vi "pco.camera_Live_Example_IMAQ.vi"() -> ()   [LabVIEW 2020]
doc: "A short program to demonstrate the fundamentals of control and image acquision with the pco.camera series. The program records a sequence of images, with \"live\" updating, until the \"StopRecording\" button is pressed. Use ctrl-H for more help on the individual controls and indicators.\n\nCopyright 2004, 2010 The Cooke Corporation."
uses:
  <userlib>/PCO LabVIEW 5.0.0/pco.camera/Camera.lvclass
  <userlib>/PCO LabVIEW 5.0.0/pco.sdk/TimingControl/TimingControl.lvlib
panel:
  in  "Trigger":bool
  in  "data_format":T1(ring)=enum."Mono16"
  out "Image":T2(plugin-control)
  out "rawImage":u16[][](array[numeric])
  in  "Image Index":u32 max=9
  out "Recorded Images":u32
  in  "TriggerMode":T3(ring)
  in  "Quit":bool
  out "Error":errorcluster {"code" format="%x"}
  in  "Stop Record":bool
  out "Recording On":bool
  in  "roiY1":u64=2 min=1 max=2160 step=1
  in  "roiX1":u64=2 min=1 max=2560 step=1
  in  "roiY0":u64=1 min=1 max=2159 step=1
  in  "roiX0":u64=1 min=1 max=2559 step=1
  out "Image Height":u64
  out "Image Width":u64
  in  "dwImgCount":u32=10 caption="Required Number of Images" max=2397
  in  "Exposure Time [s]":dbl=0.010000000000000002 min=0.0005 max=2.0 step=0.001
  # "This example demonstrates the image acquisition with one camera in ring buffer mode together with a live display of the latest images during record. After record is stopped, the images can be addressed by index.\nNote that this example will not be fail save, i.e. doesnt react on errors, just handles them forward to the end\n\nUsage:\nSelect your required image count, data format and the camera setup before you start the program.\nOnce started, the camera class will be initialized and images will be recorded and displayed automatically\nYou can stop the images by pressing stop record.\nAfter stopped, the image at the selected index will be read out\nTo finish the program click on quit application, this will force an exit of the camera class\nYou can change your required ROI after and also during the record."
  # "pco.labview"
  # "Camera Setup"
  # "Recording Control"
  # "Parameters for image readout"
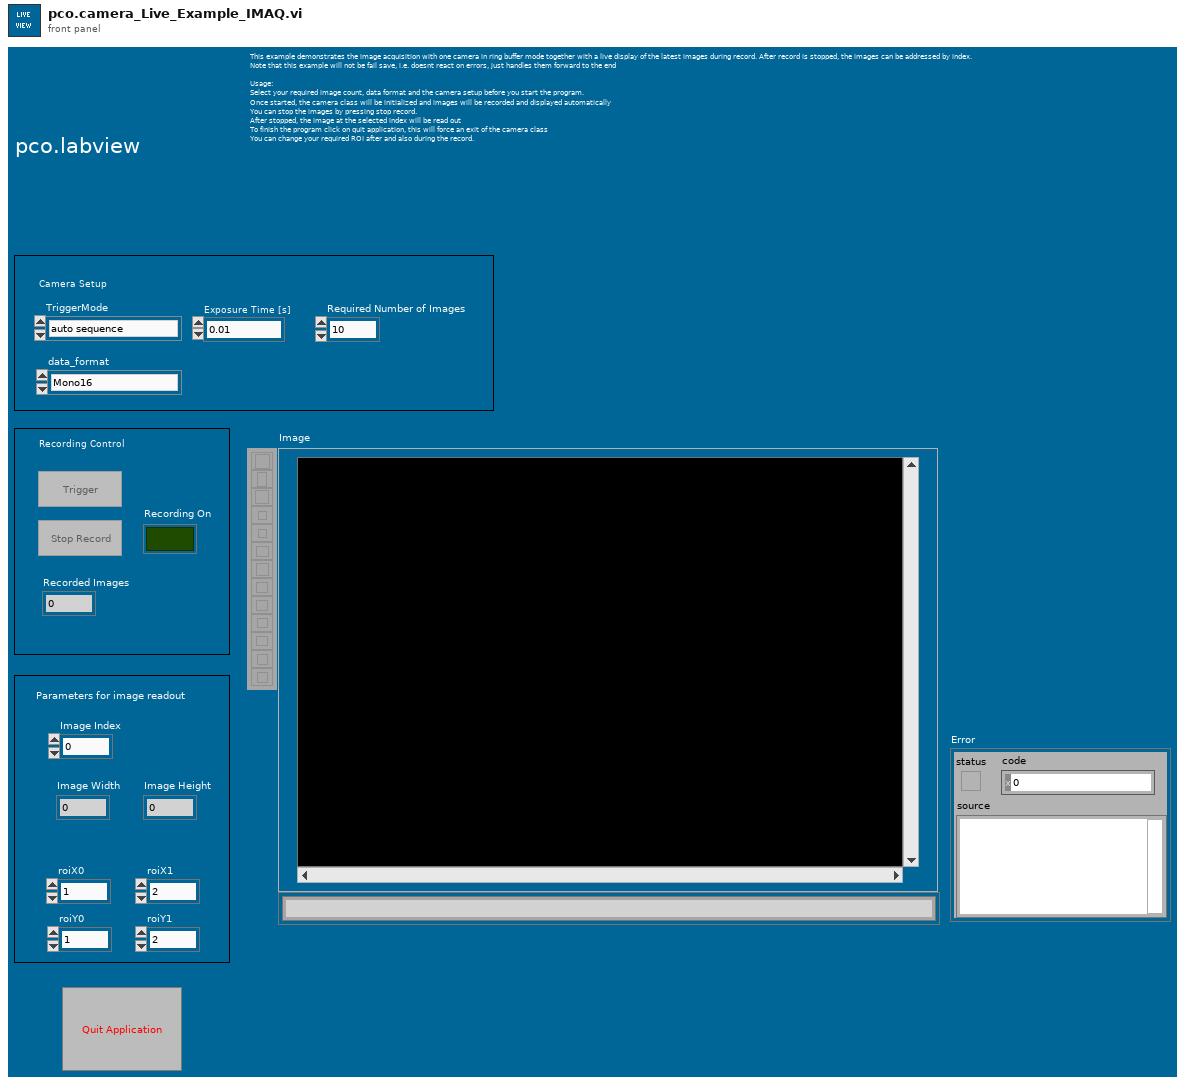
[diagram p1: front panel]
types:
  T1 = enum16{"Undefined", "Mono8", "Mono16", "BGRA8", "RGBA8", "BGRA16", "RGBA16", "CompressedMono8"}
  T2 = typedef "IMAQ Image.ctl" = refnum<image>
  T3 = enum16{"auto sequence", "software trigger", "external exposure start", "external exposure control"}
  T4 = enum16{"sequence", "sequence non blocking", "ring buffer", "fifo", "sequence_dpcore", "sequence_non_blocking_dpcore", "ring_buffer_dpcore", "fifo_dpcore", "tif", "multitif", "pcoraw", "b16", "dicom", "multidicom"}
  T5 = enum8{"Enabled", "Disabled", "Disabled and Grayed Out"}
  T6 = cluster{"serial":u32, "type":u16, "sub_type":u16, "interface_type":u16, "min_exposure_time_s":dbl, "max_exposure_time_s":dbl, "min_exposure_step_s":dbl, "min_delay_time_s":dbl, "max_delay_time_s":dbl, "min_delay_step_s":dbl, "min_width":u64, "min_height":u64, "max_width":u64, "max_height":u64, "roi_step_horz":u64, "roi_step_vert":u64, "roi_symmetric_horz":bool, "roi_symmetric_vert":bool, "has_timestamp_mode":bool, "has_timestamp_mode_ascii_only":bool, "pixelrate_vec":u32[], "has_acquire_mode":bool, "has_ext_acquire_mode":bool, "has_metadata_mode":bool, "has_ram":bool, "binning_horz_vec":u16[], "binning_vert_vec":u16[]}
  T7 = typedef "Image Type" = u32
  T8 = typedef "Camera.lvclass/binning.ctl" = cluster{"vert":u16, "horz":u16}
  T9 = cluster{"exposure_time_s":dbl, "delay_time_s":dbl, "roi":cluster{"x0":u64, "y0":u64, "x1":u64, "y1":u64}, "timestamp_mode":u16, "pixelrate":u32, "trigger_mode":u16, "acquire_mode":u16, "metadata_mode":u16, "noisefilter_mode":u16, "binning":T8}
  T10 = typedef "Color (U64)" = cluster{"Plane 3 (Blue)":u16, "Plane 2 (Green)":u16, "Plane 1 (Red)":u16, "Plane 4 (alpha)":u16}
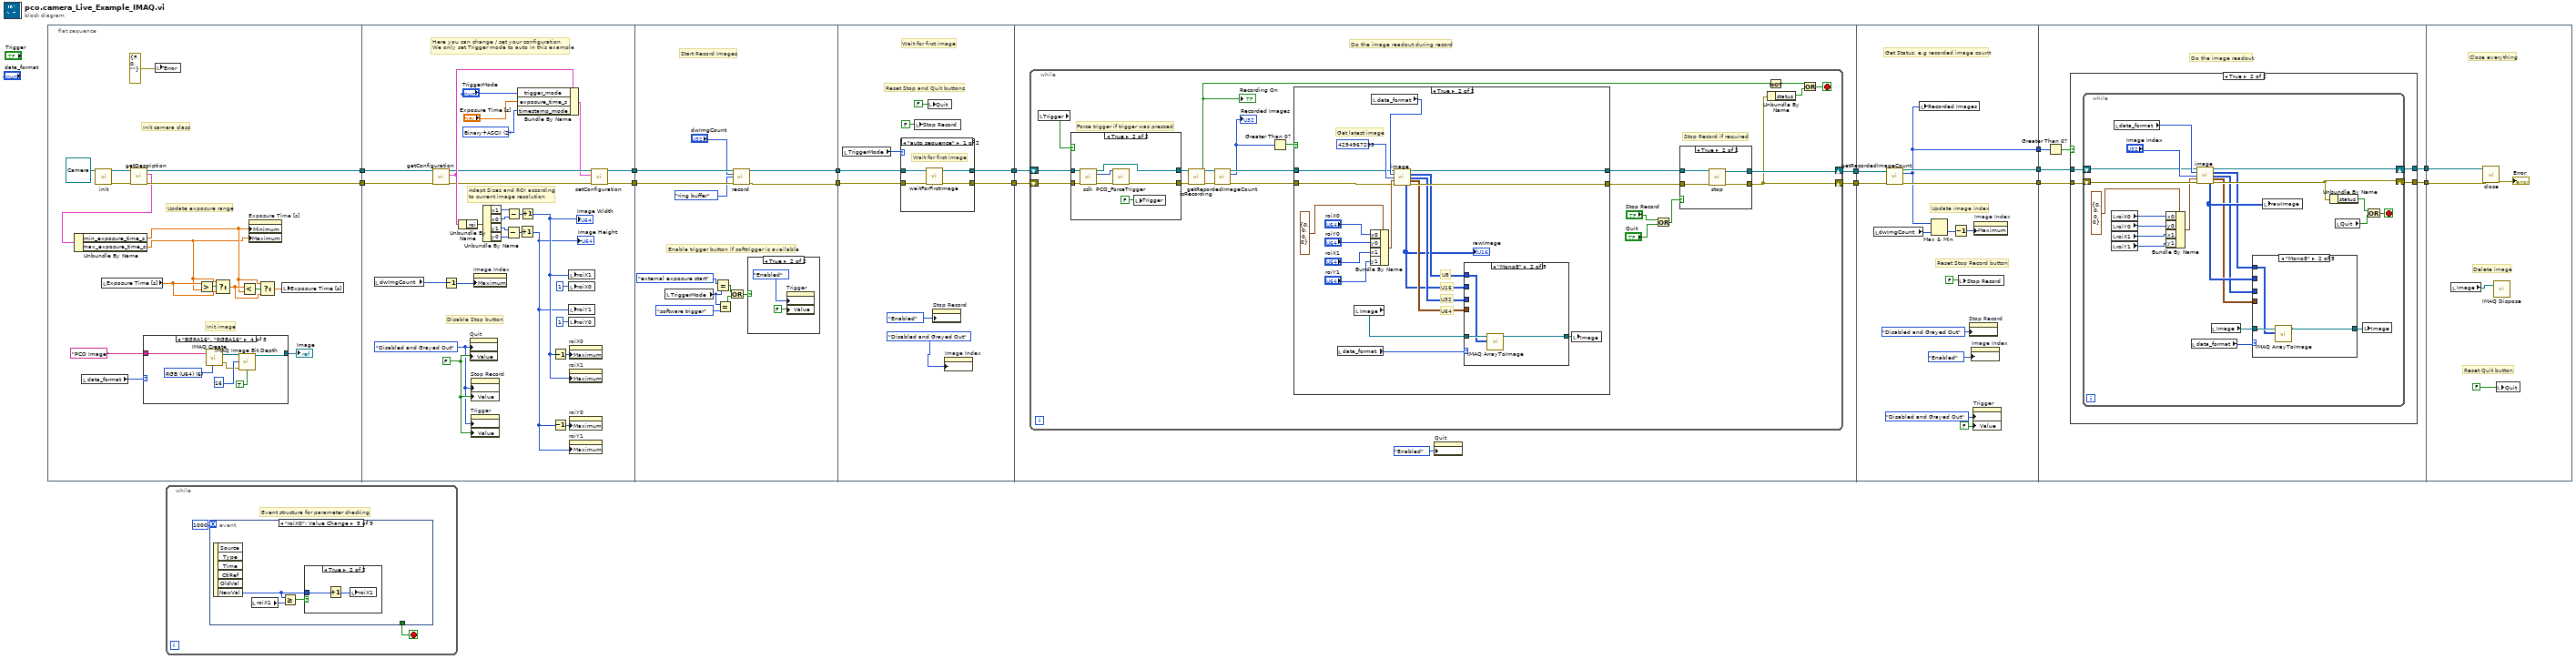
[diagram p0: block diagram]
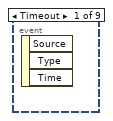
[diagram p2: hidden frame]
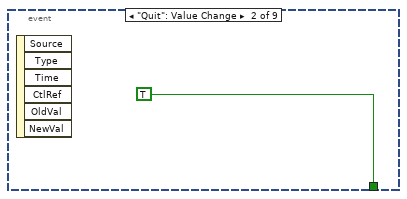
[diagram p3: hidden frame]
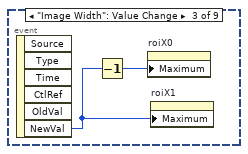
[diagram p4: hidden frame]
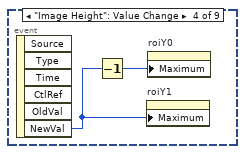
[diagram p5: hidden frame]
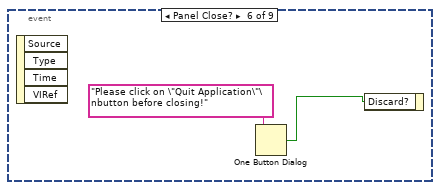
[diagram p7: hidden frame]
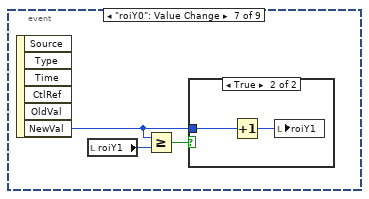
[diagram p8: hidden frame]
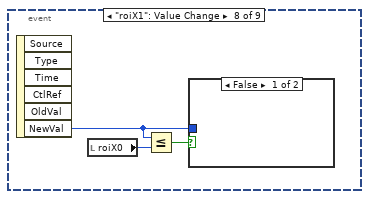
[diagram p10: hidden frame]
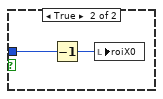
[diagram p11: hidden frame]
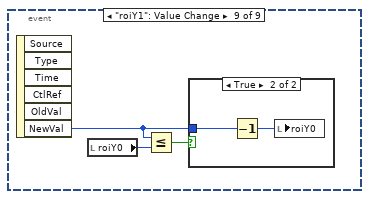
[diagram p12: hidden frame]
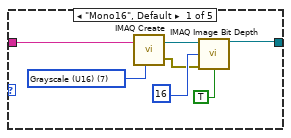
[diagram p14: hidden frame]
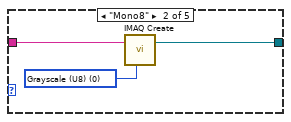
[diagram p15: hidden frame]
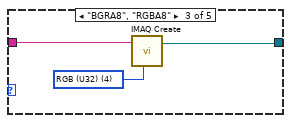
[diagram p16: hidden frame]
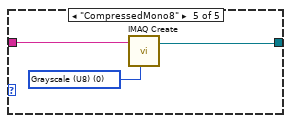
[diagram p17: hidden frame]
diagram:
  n1 = flat-sequence {
    tunnel: [w21] -> w7
    tunnel: [w20] -> w6
    tunnel: [w60] -> w15
    tunnel: [w64] -> w14
    tunnel: w7 -> [w59]
    tunnel: w6 -> [w58]
    tunnel: [w84] -> w9
    tunnel: [w85] -> w8
    tunnel: w14 -> [w95]
    tunnel: w15 -> [w94]
    tunnel: w9 -> [w102]
    tunnel: w8 -> [w103]
    tunnel: [w101] -> w13
    tunnel: [w99] -> w2
    tunnel: w13 -> [w117]
    tunnel: [w115] -> w12
    tunnel: [w114] -> w5
    tunnel: w2 -> [w113]
    tunnel: w12 -> [w200]
    tunnel: [w198] -> w11
    tunnel: w5 -> [w193]
    tunnel: [w192] -> w4
    tunnel: [w191] -> w1
    tunnel: w11 -> [w209]
    tunnel: [w208] -> w10
    tunnel: w4 -> [w207]
    tunnel: [w206] -> w3
    tunnel: w1 -> [w204]
    tunnel: w10 -> [w256]
    tunnel: w3 -> [w254]
    frame #0 {
      # "Init image"
      # "Init camera class"
      # "Update exposure range"
      n2 = local read "data_format"() -> (w16:T1)
      n3 = call-dynamic "init.vi"("Camera in"=refnum<class "Camera.lvclass"> refnum) -> ("Camera out"=w22:refnum<class "Camera.lvclass">, "error out"=w23:errorcluster)  [unwired: 8 in]
      n4 = local read "Exposure Time [s]"() -> (w31:dbl)
      n5 = call-dynamic "getDescription.vi"("error in (no error)"=w23, "Camera in"=w22) -> ("error out"=w20:errorcluster, "description"=w19:T6, "Camera out"=w21:refnum<class "Camera.lvclass">)  [unwired: 7 in]
      n6 = Unbundle By Name(w19) -> ("min_exposure_time_s"=w18:dbl, "max_exposure_time_s"=w17:dbl)
      n7 = case shown="\"BGRA16\", \"RGBA16\"" w16 {
        tunnel: "PCO Image" ("Image Name") -> [w38 w42 w44 w51 w54]
        tunnel: [w33 w40 w43 w47 w53] -> w24
        frame "Mono16", Default {
          w39 = T7 7 items=["Grayscale (U8)", "Grayscale (I16)", "Grayscale (SGL)", "Complex (CSG)", "RGB (U32)", "HSL (U32)", "RGB (U64)", "Grayscale (U16)"] ("Image Type")
          n8 = call "IMAQ Create"("Image Name"=w38, "Image Type"=w39) -> ("New Image"=w35:T2, "error out"=w34:errorcluster)  [unwired: 3 in]
          n9 = call "IMAQ Image Bit Depth"("Image"=w35, "Bit Depth (0)"=u32 16, "error in (no error)"=w34, "Get/Set Bit Depth? (Set)"=TRUE) -> ("Image Out"=w33:T2)  [unwired: 9 in, 2 out]
        }
        frame "Mono8" {
          w41 = T7 0 items=["Grayscale (U8)", "Grayscale (I16)", "Grayscale (SGL)", "Complex (CSG)", "RGB (U32)", "HSL (U32)", "RGB (U64)", "Grayscale (U16)"] ("Image Type")
          n10 = call "IMAQ Create"("Image Name"=w42, "Image Type"=w41) -> ("New Image"=w40:T2)  [unwired: 3 in, 1 out]
        }
        frame "BGRA8", "RGBA8" {
          w45 = T7 4 items=["Grayscale (U8)", "Grayscale (I16)", "Grayscale (SGL)", "Complex (CSG)", "RGB (U32)", "HSL (U32)", "RGB (U64)", "Grayscale (U16)"] ("Image Type")
          n11 = call "IMAQ Create"("Image Name"=w44, "Image Type"=w45) -> ("New Image"=w43:T2)  [unwired: 3 in, 1 out]
        }
        frame "BGRA16", "RGBA16" {
          w52 = T7 6 items=["Grayscale (U8)", "Grayscale (I16)", "Grayscale (SGL)", "Complex (CSG)", "RGB (U32)", "HSL (U32)", "RGB (U64)", "Grayscale (U16)"] ("Image Type")
          n12 = call "IMAQ Create"("Image Name"=w51, "Image Type"=w52) -> ("New Image"=w48:T2, "error out"=w46:errorcluster)  [unwired: 3 in]
          n13 = call "IMAQ Image Bit Depth"("Image"=w48, "Bit Depth (0)"=u32 16, "error in (no error)"=w46, "Get/Set Bit Depth? (Set)"=TRUE) -> ("Image Out"=w47:T2)  [unwired: 9 in, 2 out]
        }
        frame "CompressedMono8" {
          w55 = T7 0 items=["Grayscale (U8)", "Grayscale (I16)", "Grayscale (SGL)", "Complex (CSG)", "RGB (U32)", "HSL (U32)", "RGB (U64)", "Grayscale (U16)"] ("Image Type")
          n14 = call "IMAQ Create"("Image Name"=w54, "Image Type"=w55) -> ("New Image"=w53:T2)  [unwired: 3 in, 1 out]
        }
      }
      "Image" <- w24
      n15 = local write "Error"(errorcluster {"status"=FALSE, "code"=0, "source"=""} ("error IO")) -> ()
      n16 = Greater?(x=w31, y=w17) -> (0:w32:bool)
      n17 = Select(t=w17, s=w32, f=w31) -> (s? t:f=w29:dbl)
      n18 = Less?(x=w29, y=w18) -> (x < y?=w30:bool)
      n19 = property on="Exposure Time [s]" class="DigNum (strict)"("Minimum"=w18, "Maximum"=w17) -> ()  [unwired: 2 in, 2 out]
      n20 = Select(t=w18, s=w30, f=w29) -> (s? t:f=w28:dbl)
      n21 = local write "Exposure Time [s]"(w28) -> ()
    }
    frame #1 {
      w70 = u16 2 items=["OFF", "Binary", "Binary+ASCII", "ASCII"] ("wTimeStampMode")
      w57 = FALSE ("Stop")
      w56 = T5."Disabled and Grayed Out" ("Disabled")
      # "Disable Stop button"
      # "Adapt Sizes and ROI according\nto current image resolution"
      # "Here you can change / set your configuration\nWe only set Trigger mode to auto in this example"
      n22 = local read "dwImgCount"() -> (w71:u32)
      n23 = call-dynamic "getConfiguration.vi"("error in (no error)"=w58, "Camera in"=w59) -> ("error out"=w65:errorcluster, "configuration"=w76:T9, "Camera out"=w67:refnum<class "Camera.lvclass">)  [unwired: 7 in]
      n24 = Decrement(x=w71) -> (x-1=w61:u32)
      n25 = Unbundle By Name(w76) -> ("roi"=w77:cluster{"x0":u64, "y0":u64, "x1":u64, "y1":u64})
      n26 = property on="Quit" class="Bool (strict)"("DisabledEnum"=w56, "Value"=w57) -> ()  [unwired: 2 in, 2 out]
      n27 = property on="Stop Record" class="Bool (strict)"("DisabledEnum"=w56, "Value"=w57) -> ()  [unwired: 2 in, 2 out]
      n28 = property on="Trigger" class="Bool (strict)"("DisabledEnum"=w56, "Value"=w57) -> ()  [unwired: 2 in, 2 out]
      n29 = property on="Image Index" class="DigNum (strict)"("Maximum"=w61) -> ()  [unwired: 2 in, 2 out]
      n30 = Unbundle By Name(w77) -> ("x1"=w79:u64, "x0"=w78:u64, "y1"=w81:u64, "y0"=w80:u64)
      n31 = Subtract(x=w81, y=w80) -> (x-y=w83:u64)
      n32 = Subtract(x=w79, y=w78) -> (x-y=w82:u64)
      n33 = Bundle By Name(cluster=w76, "trigger_mode"="TriggerMode", "exposure_time_s"="Exposure Time [s]", "timestamp_mode"=w70) -> (w66:T9)
      n34 = Increment(x=w83) -> (x+1=w62:u64)
      "Image Height" <- w62
      n35 = Increment(x=w82) -> (x+1=w63:u64)
      "Image Width" <- w63
      n36 = Decrement(x=w63) -> (x-1=w74:u64)
      n37 = Decrement(x=w62) -> (x-1=w75:u64)
      n38 = local write "roiX1"(w63) -> ()
      n39 = local write "roiX0"(u64 1 ("roiY0")) -> ()
      n40 = local write "roiY1"(w62) -> ()
      n41 = local write "roiY0"(u64 1 ("roiY0")) -> ()
      n42 = property on="roiX0" class="DigNum (strict)"("Maximum"=w74) -> ()  [unwired: 2 in, 2 out]
      n43 = property on="roiX1" class="DigNum (strict)"("Maximum"=w63) -> ()  [unwired: 2 in, 2 out]
      n44 = property on="roiY0" class="DigNum (strict)"("Maximum"=w75) -> ()  [unwired: 2 in, 2 out]
      n45 = property on="roiY1" class="DigNum (strict)"("Maximum"=w62) -> ()  [unwired: 2 in, 2 out]
      n46 = call-dynamic "setConfiguration.vi"("error in (no error)"=w65, "configuration"=w66, "Camera in"=w67) -> ("error out"=w64:errorcluster, "Camera out"=w60:refnum<class "Camera.lvclass">)  [unwired: 7 in]
    }
    frame #2 {
      # "Enable trigger button if softtrigger is available"
      # "Start Record Images"
      n47 = local read "TriggerMode"() -> (w91:T3)
      n48 = Equal?(x=T3."external exposure start" ("TriggerMode"), y=w91) -> (x = y?=w88:bool)
      n49 = Equal?(x=w91, y=T3."software trigger" ("TriggerMode")) -> (x = y?=w87:bool)
      n50 = Or(x=w88, y=w87) -> (x .or. y?=w89:bool)
      n51 = call-dynamic "record.vi"("Camera in"=w94, "num_images"="dwImgCount", "record_mode"=T4."ring buffer", "error in (no error)"=w95) -> ("Camera out"=w85:refnum<class "Camera.lvclass">, "error out"=w84:errorcluster)  [unwired: 10 in]
      n52 = case shown="True" w89 {
        frame False {
        }
        frame True {
          n53 = property on="Trigger" class="Bool (strict)"("DisabledEnum"=T5."Enabled" ("Disabled"), "Value"=FALSE ("Trigger")) -> ()  [unwired: 2 in, 2 out]
        }
      }
    }
    frame #3 {
      # "Wait for first image"
      # "Reset Stop and Quit buttons"
      n54 = local read "TriggerMode"() -> (w98:T3)
      n55 = case shown="\"auto sequence\"" w98 {
        tunnel: w103 -> [w110 w112]
        tunnel: w102 -> [w109 w111]
        tunnel: [w108 w111] -> w101
        tunnel: [w107 w112] -> w99
        frame "auto sequence" {
          # "Wait for first image"
          n56 = call-dynamic "waitForFirstImage.vi"("error in (no error)"=w109, "Camera in"=w110) -> ("error out"=w108:errorcluster, "Camera out"=w107:refnum<class "Camera.lvclass">)  [unwired: 8 in]
        }
        frame Default {
        }
      }
      n57 = local write "Stop Record"(FALSE ("Stop Record")) -> ()
      n58 = local write "Quit"(FALSE ("Stop")) -> ()
      n59 = property on="Stop Record" class="Bool (strict)"("DisabledEnum"=T5."Enabled" ("Disabled")) -> ()  [unwired: 2 in, 2 out]
      n60 = property on="Image Index" class="DigNum (strict)"("DisabledEnum"=T5."Disabled and Grayed Out" ("Disabled")) -> ()  [unwired: 2 in, 2 out]
    }
    frame #4 {
      # "Do the image readout during record"
      n61 = while {
        shift-right: [w120] -> w115
        shift-left: w117 -> [w124]
        shift-right: [w121] -> w114
        shift-left: w113 -> [w125]
        stop <- w136 stop-if-true
        # "Force trigger if trigger was pressed"
        # "Stop Record if required"
        n62 = local read "Trigger"() -> (w126:bool)
        n63 = case shown="True" w126 {
          tunnel: w125 -> [w177 w182]
          tunnel: w124 -> [w176 w181]
          tunnel: [w177 w180] -> w123
          tunnel: [w176 w179] -> w122
          frame False {
          }
          frame True {
            n64 = call-dynamic "sdk.vi"("Camera in"=w182, "error in (no error)"=w181) -> ("Camera out"=w180:refnum<class "Camera.lvclass">, "sdk"=w183:u64, "error out"=w184:errorcluster)  [unwired: 11 in]
            n65 = call <userlib>:"PCO_ForceTrigger.vi"("error in (no error)"=w184, "ph"=w183) -> ("error out"=w179:errorcluster)  [unwired: 6 in, 3 out]
            n66 = local write "Trigger"(FALSE ("Trigger")) -> ()
          }
        }
        n67 = call-dynamic "isRecording.vi"("Camera in"=w123, "error in (no error)"=w122) -> ("Camera out"=w131:refnum<class "Camera.lvclass">, "recording"=w134:bool, "error out"=w130:errorcluster)  [unwired: 11 in]
        "Recording On" <- w134
        n68 = call-dynamic "getRecordedImageCount.vi"("Camera in"=w131, "error in (no error)"=w130) -> ("Camera out"=w128:refnum<class "Camera.lvclass">, "recorded_image_count"=w118:u32, "error out"=w129:errorcluster)  [unwired: 11 in]
        "Recorded Images" <- w118
        n69 = Greater Than 0?(x=w118) -> (x > 0?=w119:bool)
        n70 = case shown="True" w119 {
          tunnel: [w140 w155] -> w132
          tunnel: w129 -> [w140 w152]
          tunnel: w128 -> [w141 w143]
          tunnel: [w141 w142] -> w127
          frame False {
          }
          frame True {
            # "U64"
            # "U32"
            # "U8"
            # "U16"
            # "Get latest image"
            n71 = local read "data_format"() -> (w144:T1)
            n72 = local read "Image"() -> (w149:T2)
            n73 = Bundle By Name(cluster=cluster{"x0":u64, "y0":u64, "x1":u64, "y1":u64} {"x0"=0, "y0"=0, "x1"=0, "y1"=0} ("roi"), "x0"="roiX0", "y0"="roiY0", "x1"="roiX1", "y1"="roiY1") -> (w156:cluster{"x0":u64, "y0":u64, "x1":u64, "y1":u64})
            n74 = local read "data_format"() -> (w151:T1)
            n75 = call-dynamic "image.vi"("Camera in"=w143, "data_format"=w151, "image_index"=u32 4294967295 ("dwImgIdx"), "roi"=w156, "error in (no error)"=w152) -> ("Camera out"=w142:refnum<class "Camera.lvclass">, "image (U8)"=w146:u8[][], "image (U32)"=w147:u32[][], "image (U64)"=w148:T10[][], "raw_image (U16)"=w145:u16[][], "error out"=w155:errorcluster)  [unwired: 3 in, 2 out]
            "rawImage" <- w145
            n76 = case shown="\"Mono8\"" w144 {
              tunnel: w149 -> [w163 w166 w169 w172 w175]
              tunnel: [w161 w164 w168 w170 w174] -> w150
              tunnel: w148 -> [_ _ _ w171 _]
              tunnel: w147 -> [_ _ w167 _ _]
              tunnel: w146 -> [_ w165 _ _ w173]
              tunnel: w145 -> [w162 _ _ _ _]
              frame "Mono16", Default {
                n77 = call "IMAQ ArrayToImage"("Image Pixels (U16)"=w162, "Image"=w163) -> ("Image Out"=w161:T2)  [unwired: 8 in, 1 out]
              }
              frame "Mono8" {
                n78 = call "IMAQ ArrayToImage"("Image Pixels (U8)"=w165, "Image"=w166) -> ("Image Out"=w164:T2)  [unwired: 8 in, 1 out]
              }
              frame "BGRA8", "RGBA8" {
                n79 = call "IMAQ ArrayToColorImage"("Image Pixels (U32)"=w167, "Image"=w169) -> ("Image Out"=w168:T2)  [unwired: 3 in, 1 out]
              }
              frame "BGRA16", "RGBA16" {
                n80 = call "IMAQ ArrayToColorImage"("Image"=w172, "Image Pixels (U64)"=w171) -> ("Image Out"=w170:T2)  [unwired: 3 in, 1 out]
              }
              frame "CompressedMono8" {
                n81 = call "IMAQ ArrayToImage"("Image Pixels (U8)"=w173, "Image"=w175) -> ("Image Out"=w174:T2)  [unwired: 8 in, 1 out]
              }
            }
            n82 = local write "Image"(w150) -> ()
          }
        }
        n83 = Or(x="Stop Record", y="Quit") -> (x .or. y?=w137:bool)
        n84 = case shown="True" w137 {
          tunnel: w132 -> [w186 w187]
          tunnel: [w185 w189] -> w121
          tunnel: [w186 w190] -> w120
          tunnel: w127 -> [w185 w188]
          frame False {
          }
          frame True {
            n85 = call-dynamic "stop.vi"("error in (no error)"=w187, "Camera in"=w188) -> ("error out"=w190:errorcluster, "Camera out"=w189:refnum<class "Camera.lvclass">)  [unwired: 8 in]
          }
        }
        n86 = Unbundle By Name(w120) -> ("status"=w135:bool)
        n87 = Not(x=w134) -> (.not. x?=w133:bool)
        n88 = Or(x=w133, y=w135) -> (x .or. y?=w136:bool)
      }
      n89 = property on="Quit" class="Bool (strict)"("DisabledEnum"=T5."Enabled" ("Disabled")) -> ()  [unwired: 2 in, 2 out]
    }
    frame #5 {
      # "Update image index"
      # "Reset Stop Record button"
      # "Get Status, e.g recorded image count"
      n90 = local read "dwImgCount"() -> (w199:u32)
      n91 = call-dynamic "getRecordedImageCount.vi"("Camera in"=w193, "error in (no error)"=w200) -> ("Camera out"=w192:refnum<class "Camera.lvclass">, "recorded_image_count"=w191:u32, "error out"=w198:errorcluster)  [unwired: 11 in]
      n92 = local write "Recorded Images"(w191) -> ()
      n93 = Max & Min(x=w191, y=w199) -> (min(x,y)=w201:u32)  [unwired: 1 out]
      n94 = Decrement(x=w201) -> (x-1=w196:u32)
      n95 = local write "Stop Record"(FALSE ("Stop Record")) -> ()
      n96 = property on="Stop Record" class="Bool (strict)"("DisabledEnum"=T5."Disabled and Grayed Out" ("Disabled")) -> ()  [unwired: 2 in, 2 out]
      n97 = property on="Image Index" class="DigNum (strict)"("DisabledEnum"=T5."Enabled" ("Disabled")) -> ()  [unwired: 2 in, 2 out]
      n98 = property on="Trigger" class="Bool (strict)"("DisabledEnum"=T5."Disabled and Grayed Out" ("Disabled"), "Value"=FALSE ("Trigger")) -> ()  [unwired: 2 in, 2 out]
      n99 = property on="Image Index" class="DigNum (strict)"("Maximum"=w196) -> ()  [unwired: 2 in, 2 out]
    }
    frame #6 {
      # "Do the image readout"
      n100 = Greater Than 0?(x=w204) -> (x > 0?=w205:bool)
      n101 = case shown="True" w205 {
        tunnel: w209 -> [w210 w215]
        tunnel: [w210 w214] -> w208
        tunnel: w207 -> [w211 w213]
        tunnel: [w211 w212] -> w206
        frame False {
        }
        frame True {
          n102 = while {
            shift-right: [w229] -> w214
            shift-left: w215 -> [w237]
            shift-right: [w216] -> w212
            shift-left: w213 -> [w217]
            stop <- w231 stop-if-true
            n103 = local read "roiX0"() -> (w227:u64)
            n104 = local read "roiY0"() -> (w228:u64)
            n105 = local read "roiX1"() -> (w235:u64)
            n106 = local read "roiY1"() -> (w234:u64)
            n107 = local read "data_format"() -> (w225:T1)
            n108 = Bundle By Name(cluster=cluster{"x0":u64, "y0":u64, "x1":u64, "y1":u64} {"x0"=0, "y0"=0, "x1"=0, "y1"=0} ("roi"), "x0"=w227, "y0"=w228, "x1"=w235, "y1"=w234) -> (w236:cluster{"x0":u64, "y0":u64, "x1":u64, "y1":u64})
            n109 = local read "data_format"() -> (w218:T1)
            n110 = call-dynamic "image.vi"("Camera in"=w217, "data_format"=w225, "image_index"="Image Index", "roi"=w236, "error in (no error)"=w237) -> ("Camera out"=w216:refnum<class "Camera.lvclass">, "image (U8)"=w221:u8[][], "image (U32)"=w220:u32[][], "image (U64)"=w219:T10[][], "raw_image (U16)"=w222:u16[][], "error out"=w229:errorcluster)  [unwired: 3 in, 2 out]
            n111 = local read "Image"() -> (w223:T2)
            n112 = case shown="\"Mono8\"" w218 {
              tunnel: w223 -> [w240 w243 w246 w249 w252]
              tunnel: [w238 w241 w245 w247 w251] -> w224
              tunnel: w219 -> [_ _ _ w248 _]
              tunnel: w220 -> [_ _ w244 _ _]
              tunnel: w221 -> [_ w242 _ _ w250]
              tunnel: w222 -> [w239 _ _ _ _]
              frame "Mono16", Default {
                n113 = call "IMAQ ArrayToImage"("Image Pixels (U16)"=w239, "Image"=w240) -> ("Image Out"=w238:T2)  [unwired: 8 in, 1 out]
              }
              frame "Mono8" {
                n114 = call "IMAQ ArrayToImage"("Image Pixels (U8)"=w242, "Image"=w243) -> ("Image Out"=w241:T2)  [unwired: 8 in, 1 out]
              }
              frame "BGRA8", "RGBA8" {
                n115 = call "IMAQ ArrayToColorImage"("Image Pixels (U32)"=w244, "Image"=w246) -> ("Image Out"=w245:T2)  [unwired: 3 in, 1 out]
              }
              frame "BGRA16", "RGBA16" {
                n116 = call "IMAQ ArrayToColorImage"("Image"=w249, "Image Pixels (U64)"=w248) -> ("Image Out"=w247:T2)  [unwired: 3 in, 1 out]
              }
              frame "CompressedMono8" {
                n117 = call "IMAQ ArrayToImage"("Image Pixels (U8)"=w250, "Image"=w252) -> ("Image Out"=w251:T2)  [unwired: 8 in, 1 out]
              }
            }
            n118 = local write "rawImage"(w222) -> ()
            n119 = Unbundle By Name(w229) -> ("status"=w232:bool)
            n120 = local read "Quit"() -> (w233:bool)
            n121 = local write "Image"(w224) -> ()
            n122 = Or(x=w232, y=w233) -> (x .or. y?=w231:bool)
          }
        }
      }
    }
    frame #7 {
      # "Delete image"
      # "Close everything"
      # "Reset Quit button"
      n123 = local read "Image"() -> (w253:T2)
      n124 = call-dynamic "close.vi"("error in (no error)"=w256, "Camera in"=w254) -> ("error out"=→"Error":errorcluster)  [unwired: 9 in]
      n125 = call "IMAQ Dispose"("Image"=w253) -> ()  [unwired: 5 in, 1 out]
      n126 = local write "Quit"(FALSE ("Stop Record")) -> ()
    }
  }
  n127 = while {
    stop <- w258 stop-if-true
    # "Event structure for parameter checking"
    n128 = event shown="[4] \"roiX0\": Value Change" {
      selector: _ -> [_ _ _ _ _ _ _ _ _]
      dyn-events: _ -> [_ _ _ _ _ _ _ _ _]
      timeout: 1000 -> [_ _ _ _ _ _ _ _ _]
      tunnel: [_ TRUE _ _ _ _ _ _ _] -> w258
      event Timeout {
        n129 = event-data() -> ()  [unwired: 1 in, 3 out]
      }
      event "Quit": Value Change {
        n130 = event-data() -> ()  [unwired: 1 in, 6 out]
      }
      event "Image Width": Value Change {
        n131 = event-data() -> ("NewVal"=w261:u64)  [unwired: 1 in, 5 out]
        n132 = Decrement(x=w261) -> (x-1=w262:u64)
        n133 = property on="roiX0" class="DigNum (strict)"("Maximum"=w262) -> ()  [unwired: 2 in, 2 out]
        n134 = property on="roiX1" class="DigNum (strict)"("Maximum"=w261) -> ()  [unwired: 2 in, 2 out]
      }
      event "Image Height": Value Change {
        n135 = event-data() -> ("NewVal"=w263:u64)  [unwired: 1 in, 5 out]
        n136 = Decrement(x=w263) -> (x-1=w264:u64)
        n137 = property on="roiY1" class="DigNum (strict)"("Maximum"=w263) -> ()  [unwired: 2 in, 2 out]
        n138 = property on="roiY0" class="DigNum (strict)"("Maximum"=w264) -> ()  [unwired: 2 in, 2 out]
      }
      event "roiX0": Value Change {
        n139 = event-data() -> ("NewVal"=w265:u64)  [unwired: 1 in, 5 out]
        n140 = local read "roiX1"() -> (w267:u64)
        n141 = Greater Or Equal?(x=w265, y=w267) -> (x >= y?=w266:bool)
        n142 = case shown="True" w266 {
          tunnel: w265 -> [_ w269]
          frame False {
          }
          frame True {
            n143 = Increment(x=w269) -> (x+1=w268:u64)
            n144 = local write "roiX1"(w268) -> ()
          }
        }
      }
      event Panel Close? {
        n145 = event-data() -> ()  [unwired: 1 in, 4 out]
        n146 = One Button Dialog(message="Please click on \"Quit Application\"\nbutton before closing!") -> (true=w270:bool)  [unwired: 1 in]
        n147 = event-data("Discard?"=w270) -> ()  [unwired: 1 in, 1 out]
      }
      event "roiY0": Value Change {
        n148 = event-data() -> ("NewVal"=w272:u64)  [unwired: 1 in, 5 out]
        n149 = local read "roiY1"() -> (w274:u64)
        n150 = Greater Or Equal?(x=w272, y=w274) -> (x >= y?=w273:bool)
        n151 = case shown="True" w273 {
          tunnel: w272 -> [_ w276]
          frame False {
          }
          frame True {
            n152 = Increment(x=w276) -> (x+1=w275:u64)
            n153 = local write "roiY1"(w275) -> ()
          }
        }
      }
      event "roiX1": Value Change {
        n154 = event-data() -> ("NewVal"=w277:u64)  [unwired: 1 in, 5 out]
        n155 = local read "roiX0"() -> (w279:u64)
        n156 = Less Or Equal?(x=w277, y=w279) -> (x <= y?=w278:bool)
        n157 = case shown="False" w278 {
          tunnel: w277 -> [_ w281]
          frame False {
          }
          frame True {
            n158 = Decrement(x=w281) -> (x-1=w280:u64)
            n159 = local write "roiX0"(w280) -> ()
          }
        }
      }
      event "roiY1": Value Change {
        n160 = event-data() -> ("NewVal"=w282:u64)  [unwired: 1 in, 5 out]
        n161 = local read "roiY0"() -> (w284:u64)
        n162 = Less Or Equal?(x=w282, y=w284) -> (x <= y?=w283:bool)
        n163 = case shown="True" w283 {
          tunnel: w282 -> [_ w286]
          frame False {
          }
          frame True {
            n164 = Decrement(x=w286) -> (x-1=w285:u64)
            n165 = local write "roiY0"(w285) -> ()
          }
        }
      }
    }
  }
